vi "ReadWrite.ProcessData.Commit.vi"(8 "error in":errorcluster, 11 "ReadWrite in":refnum<class "ReadWrite.lvclass">) -> (0 "error out":errorcluster, 3 "ReadWrite out":refnum<class "ReadWrite.lvclass">)   [LabVIEW 2026, in "Data Access Engine (Express).lvlib" / "ReadWrite.lvclass"]
uses:
  ReadWrite.lvclass
  ReadWrite.lvclass/ReadWrite.ctl
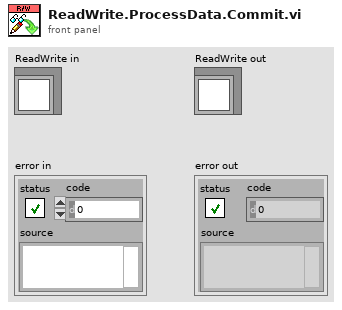
[diagram p1: front panel]
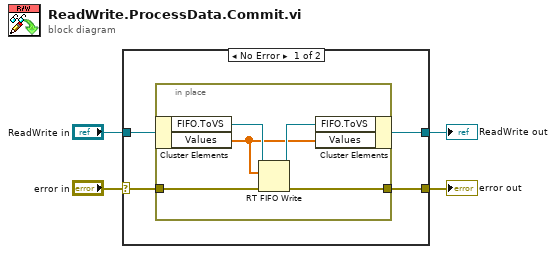
[diagram p0: block diagram]
diagram:
  n1 = case shown="No Error" "error in" {
    selector: "error in" -> [w8 w14]
    tunnel: [w7 w14] -> w3
    tunnel: [w5 w15] -> w1
    tunnel: "ReadWrite in" -> [w6 w15]
    frame No Error {
      n2 = in-place {
        in-place-border: w8 -> [w10]
        in-place-border: [w11] -> w7
        n3 = in-place-cluster #1(w6) -> ("FIFO.ToVS"=w13:refnum<k33>, "Values"=w9:dbl[])
        n4 = RT FIFO Write(0:w13, 1:w9, 3:w10) -> (8:w12:refnum<k33>, 11:w11:errorcluster)  [unwired: 2 in, 2 out]
        n5 = in-place-cluster #1("FIFO.ToVS"=w12, "Values"=w9) -> (w5:refnum<class "ReadWrite.lvclass">)
      }
    }
    frame Error {
    }
  }
  "error out" <- w3
  "ReadWrite out" <- w1
